vi "IkiGetPosition.vi"(6 "error in (no error)":errorcluster, 9 "connection ID":refnum<k5>) -> (0 "error out":errorcluster, 3 "connection ID out":refnum<k5>, 4 "Y":dbl, 5 "X":dbl)   [LabVIEW 2009]
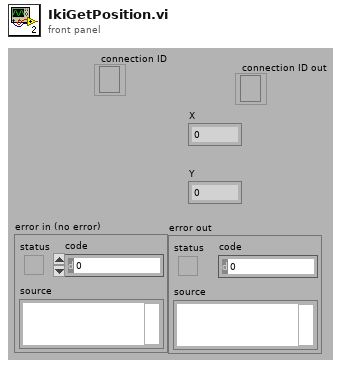
[diagram p1: front panel]
types:
  T1 = enum16{"Standard", "Buffered", "CRLF", "Immediate"}
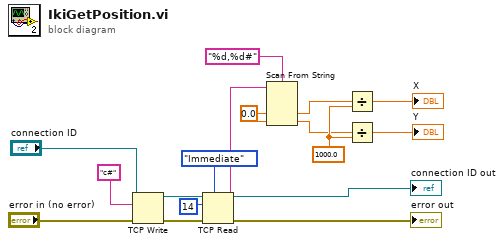
[diagram p0: block diagram]
diagram:
  w12 = 1000.0 ("y")
  w8 = 0.0 ("valeur par défaut1")
  n1 = TCP Write(connection ID="connection ID", data in="c#" ("données d'entrée"), error in (no error)="error in (no error)") -> (connection ID out=w3:refnum<k5>, error out=w4:errorcluster)  [unwired: 1 in, 1 out]
  n2 = TCP Read(connection ID=w3, bytes to read=14 ("octets à lire"), error in (no error)=w4, 7:T1."Immediate" ("mode (standard)")) -> (connection ID out=→"connection ID out":refnum<k5>, data out=w9:string, error out=→"error out":errorcluster)  [unwired: 1 in]
  n3 = Scan From String(format string="%d,%d#" ("chaîne de format"), input string=w9, default 1=w8, default 2=w8) -> (output 1=w10:dbl, output 2=w11:dbl)  [unwired: 2 in, 3 out]
  n4 = Divide(x=w10, y=w12) -> (x/y=→"X":dbl)
  n5 = Divide(x=w11, y=w12) -> (x/y=→"Y":dbl)
